vi "SetTorWfmDataSetId.vi"(9 "DataSetName":string, 10 "DataSetIds":variant, 11 "props in":T1[](array[typedef])) -> (3 "props out":T1[](array[typedef]))   [LabVIEW 2017, in "McsaDataEventCreator.lvlib"]
uses:
  <vilib>/addons/InsightCM/Devices/Shared/Mcsa/McsaDataEventCreator/McsaDataEventCreator.lvlib
  <vilib>/addons/InsightCM/MessageBus/Base/controls/KeyValuePair.ctl
  <vilib>/addons/InsightCM/Devices/Shared/Mcsa/McsaDataEventCreator/controls/DataSetType.ctl
  <vilib>/addons/InsightCM/Utilities/PropertyHelpers/PropertyHelpers.lvlib
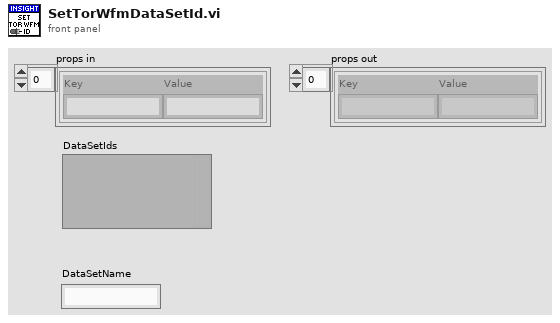
[diagram p1: front panel]
types:
  T1 = typedef "KeyValuePair.ctl" = cluster{"Key":string, "Value":string}
  T2 = typedef "McsaDataEventCreator.lvlib/DataSetType.ctl" = enum16{"Waveform", "MCSAFFT", "TorqueWFM"}
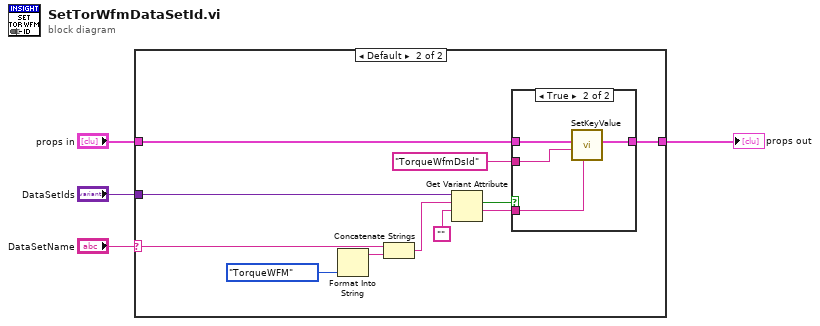
[diagram p0: block diagram]
diagram:
  n1 = case shown="Default" "DataSetName" {
    selector: "DataSetName" -> [_ w9]
    tunnel: [w5 w13] -> w4
    tunnel: "props in" -> [w5 w14]
    tunnel: "DataSetIds" -> [_ w16]
    frame "" {
    }
    frame Default {
      n2 = Format Into String(DataSetType."TorqueWFM" ("DataSetType")) -> (resulting string=w8:string)  [unwired: 3 in, 1 out]
      n3 = Concatenate Strings(w9, w8) -> (w7:string)
      n4 = Get Variant Attribute(Variant=w16, name=w7, default value (empty Variant)="") -> (found=w10:bool, value=w11:string)  [unwired: 1 in, 2 out]
      n5 = case shown="True" w10 {
        tunnel: w14 -> [w17 w21]
        tunnel: [w17 w20] -> w13
        tunnel: "TorqueWfmDsId" -> [_ w19]
        tunnel: w11 -> [_ w18]
        frame False {
        }
        frame True {
          n6 = call <vilib>:"SetKeyValue.vi"("value"=w18, "key"=w19, "key value pairs"=w21) -> ("key value pairs out"=w20:T1[])  [unwired: 8 in]
        }
      }
    }
  }
  "props out" <- w4
